vi "Close.vi"(8 "error in (no error)":errorcluster, 11 "Inst.TSL210 in":refnum<class "Inst.TSL210.lvclass">) -> (0 "error out":errorcluster, 3 "Inst.TSL210 out":refnum<class "Inst.TSL210.lvclass">)   [LabVIEW 2019, in "Inst.TSL210.lvclass"]
uses:
  Inst.TSL210.lvclass
  C:/Program Files (x86)/National Instruments/LabVIEW 2019/user.lib/LevyLab/Instrument Framework/SMOs/Instrument/Instrument.lvclass
  <userlib>/LevyLab/Instrument Framework/Instrument Types/VSource/Instrument.VSource.lvclass
  <userlib>/LevyLab/Instrument Framework/SMOs/Instrument/Instrument.lvclass
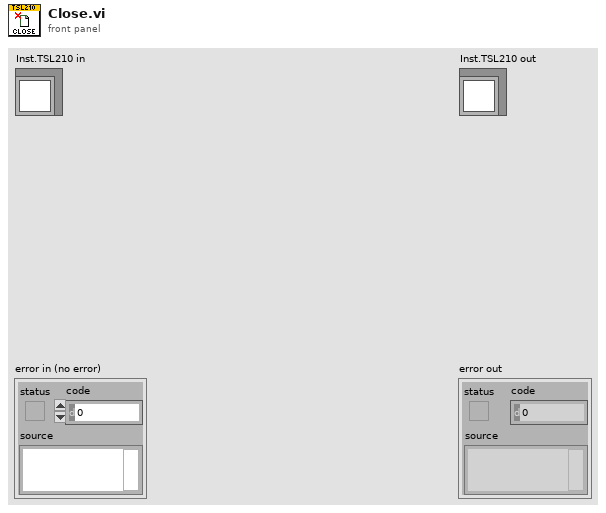
[diagram p1: front panel]
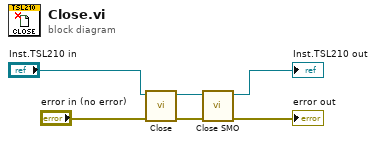
[diagram p0: block diagram]
diagram:
  n1 = call-parent "Close.vi"("error in (no error)"="error in (no error)", "Instrument in"="Inst.TSL210 in") -> ("error out"=w4:errorcluster, "Instrument out"=w3:refnum<class "Inst.TSL210.lvclass">)  [unwired: 8 in]
  n2 = call <userlib>:"Close SMO.vi"("error in (no error)"=w4, "Instrument in"=w3) -> ("error out"=→"error out":errorcluster, "Instrument out"=→"Inst.TSL210 out":refnum<class "Inst.TSL210.lvclass">)  [unwired: 8 in]
